vi "Configure List Operation.vi"(0 "VISA resource name":refnum<visa-resource-name>, 1 "Number of Steps(1)":dbl=1.0 format="%.2f", 2 "Steps Count(2)":dbl=2.0, 5 "List Mode(0:Continuous)":u16(ring) items=["Continuous", "Step"], 7 "List Repeat Mode(0:Once)":u16(ring) items=["Once", "Repeat  "], 9 "List Operation(0:Voltage)":u16(ring) items=["Voltage", "Current"], 11 "error in (no error)":errorcluster, 12 "Manual Range(0.00)":dbl format="%.2f", 13 "Unit(V)":u16(ring) items=["V", "mV", "A", "mA"]) -> (4 "VISA resource name out":refnum<visa-resource-name>, 15 "error out":errorcluster)   [LabVIEW 2021, in "Keithley 2200 Series.lvlib"]
doc: "Configure list operation.\n\nNote: This VI should be set first before all other list operation configurations."
uses:
  <instrlib>/Keithley 2200 Series/Keithley 2200 Series.lvlib
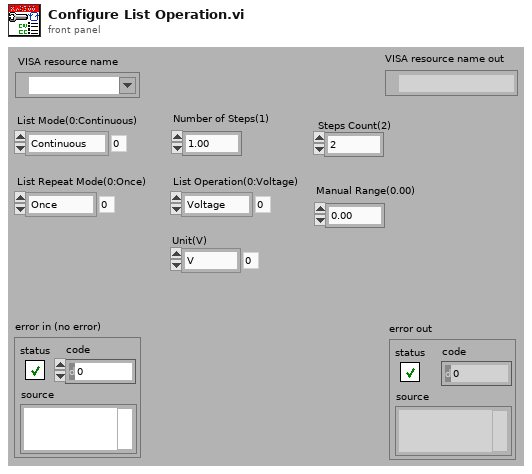
[diagram p1: front panel]
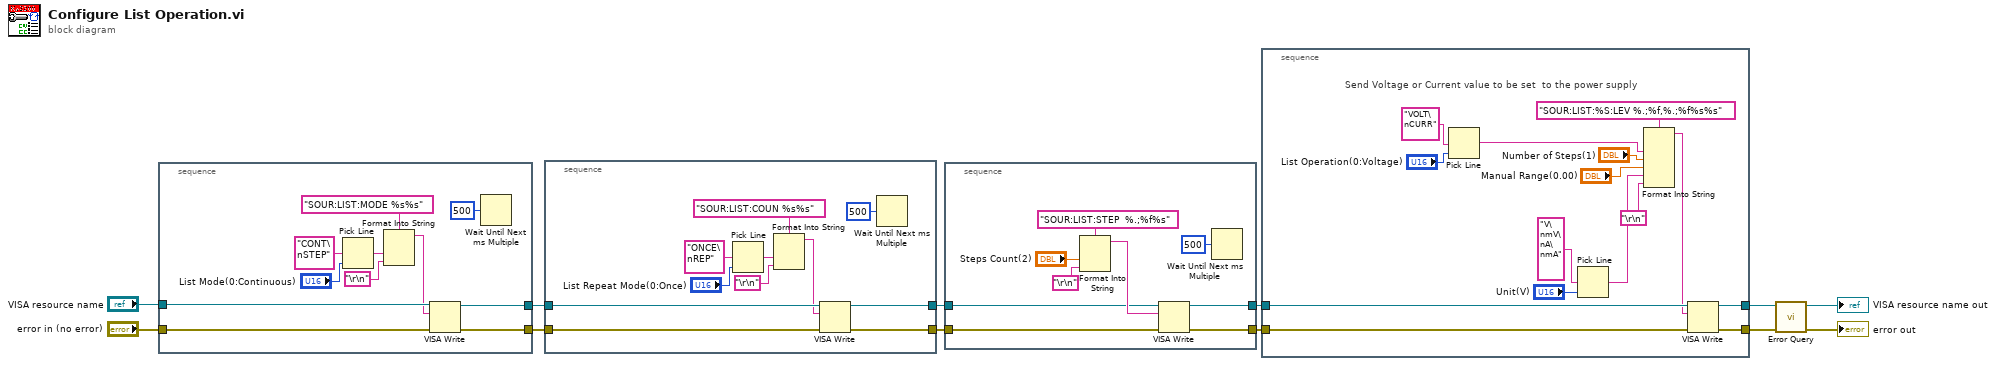
[diagram p0: block diagram]
diagram:
  n1 = stacked-sequence {
    tunnel: "error in (no error)" -> [w23]
    tunnel: "VISA resource name" -> [w22]
    tunnel: [w16] -> w10
    tunnel: [w15] -> w9
    frame #0 {
      n2 = Pick Line(multi-line string="CONT\nSTEP", line index="List Mode(0:Continuous)") -> (output string=w17:string)  [unwired: 1 out]
      n3 = Format Into String(format string="SOUR:LIST:MODE %s%s", w17, "\r\n" ("End of Line Constant")) -> (resulting string=w14:string)  [unwired: 2 in, 1 out]
      n4 = VISA Write(VISA resource name=w22, write buffer=w14, error in (no error)=w23) -> (VISA resource name out=w16:refnum<visa-resource-name>, error out=w15:errorcluster)  [unwired: 1 out]
      n5 = Wait Until Next ms Multiple(millisecond multiple=u32 500 ("Programmable Delay in ms")) -> ()  [unwired: 1 out]
    }
  }
  n6 = stacked-sequence {
    tunnel: w10 -> [w34]
    tunnel: w9 -> [w33]
    tunnel: [w32] -> w4
    tunnel: [w31] -> w3
    frame #0 {
      n7 = Pick Line(multi-line string="ONCE\nREP", line index="List Repeat Mode(0:Once)") -> (output string=w26:string)  [unwired: 1 out]
      n8 = Format Into String(format string="SOUR:LIST:COUN %s%s", w26, "\r\n" ("End of Line Constant")) -> (resulting string=w25:string)  [unwired: 2 in, 1 out]
      n9 = VISA Write(VISA resource name=w34, write buffer=w25, error in (no error)=w33) -> (VISA resource name out=w32:refnum<visa-resource-name>, error out=w31:errorcluster)  [unwired: 1 out]
      n10 = Wait Until Next ms Multiple(millisecond multiple=u32 500 ("Programmable Delay in ms")) -> ()  [unwired: 1 out]
    }
  }
  n11 = stacked-sequence {
    tunnel: w4 -> [w39]
    tunnel: w3 -> [w38]
    tunnel: [w37] -> w2
    tunnel: [w36] -> w1
    frame #0 {
      n12 = Format Into String(format string="SOUR:LIST:STEP  %.;%f%s", "Steps Count(2)", "\r\n" ("End of Line Constant")) -> (resulting string=w41:string)  [unwired: 2 in, 1 out]
      n13 = VISA Write(VISA resource name=w39, write buffer=w41, error in (no error)=w38) -> (VISA resource name out=w37:refnum<visa-resource-name>, error out=w36:errorcluster)  [unwired: 1 out]
      n14 = Wait Until Next ms Multiple(millisecond multiple=u32 500 ("Programmable Delay in ms")) -> ()  [unwired: 1 out]
    }
  }
  n15 = stacked-sequence {
    tunnel: [w58] -> w8
    tunnel: [w57] -> w7
    tunnel: w2 -> [w47]
    tunnel: w1 -> [w46]
    frame #0 {
      # "Send Voltage or Current value to be set  to the power supply"
      n16 = Pick Line(multi-line string="VOLT\nCURR" ("format string"), line index="List Operation(0:Voltage)") -> (output string=w53:string)  [unwired: 1 out]
      n17 = Pick Line(multi-line string="V\nmV\nA\nmA", line index="Unit(V)") -> (output string=w49:string)  [unwired: 1 out]
      n18 = Format Into String(format string="SOUR:LIST:%S:LEV %.;%f,%.;%f%s%s", w53, "Number of Steps(1)", "Manual Range(0.00)", w49, "\r\n" ("End of Line Constant")) -> (resulting string=w44:string)  [unwired: 2 in, 1 out]
      n19 = VISA Write(VISA resource name=w47, write buffer=w44, error in (no error)=w46) -> (VISA resource name out=w58:refnum<visa-resource-name>, error out=w57:errorcluster)  [unwired: 1 out]
    }
  }
  n20 = call <instrlib>:"Error Query.vi"("error in (no error)"=w7, "VISA resource name"=w8) -> ("error out"=→"error out":errorcluster, "VISA resource name out"=→"VISA resource name out":refnum<visa-resource-name>)  [unwired: 8 out]
